vi "Find Highlights.vi"(10 "Type":enum16{"added", "missing"}(ring), 11 "String":string) -> (3 "Sections":T1(array[cluster]))   [LabVIEW 2020]
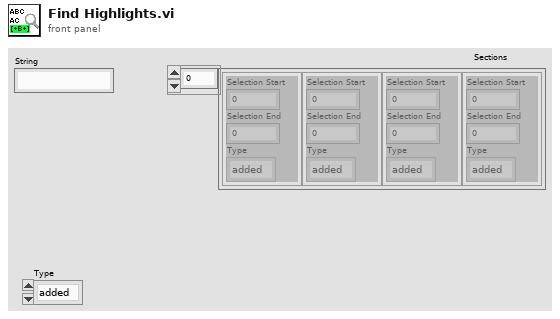
[diagram p1: front panel]
types:
  T1 = cluster{"Selection Start":u32, "Selection End":u32, "Type":enum16{"added", "missing"}}[]
  T2 = cluster{"Selection Start":u32, "Selection End":u32, "Type":enum16{"added", "missing"}}
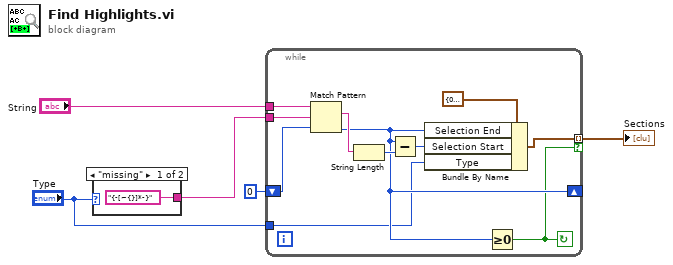
[diagram p0: block diagram]
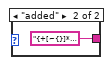
[diagram p2: hidden frame]
diagram:
  n1 = case shown="\"missing\"" "Type" {
    tunnel: ["{-[~{}]*-}" ("regular expression") "{+[~{}]*+}" ("regular expression")] -> w4
    frame "missing" {
    }
    frame "added" {
    }
  }
  n2 = while {
    tunnel: "String" -> [w18]
    tunnel: w4 -> [w17]
    tunnel: [w12] -> w3 mode=indexing if=w9
    shift-right: [w11] -> _
    shift-left: 0 ("offset past match") -> [w10]
    tunnel: "Type" -> [w8]
    stop <- w9 continue-if-true
    n3 = Match Pattern(string=w18, regular expression=w17, offset (0)=w10) -> (match substring=w16:string, offset past match=w11:i32)  [unwired: 2 out]
    n4 = String Length(string=w16) -> (length=w14:i32)
    n5 = Subtract(x=w11, y=w14) -> (x-y=w13:i32)
    n6 = Bundle By Name(cluster=T2 {"Selection Start"=0, "Selection End"=0, "Type"=enum."added"} ("Sections"), "Selection End"=w11, "Selection Start"=w13, "Type"=w8) -> (w12:T2)
    n7 = Greater Or Equal To 0?(x=w11) -> (x >= 0?=w9:bool)
  }
  "Sections" <- w3
